vi "FPGA_main.vi"() -> ()   [LabVIEW 2016]
uses:
  <vilib>/rvi/Emulation/niFpgaGetClockAttributes.vi
  <vilib>/rvi/Emulation/niFpgaSctlEmulationGetInTimedLoop.vi
  <vilib>/rvi/Emulation/niFpgaEmulationReportErrorSimple.vi
  <vilib>/rvi/eio/common/nirviEmuTemplateMethod_errors.vi
  <vilib>/rvi/Emulation/niFpgaCriticalErrorInLSC.vi
  <vilib>/eio/EIONode/EIONode.xnode
panel:
  in  "L1":i32=52
  in  "H1":i32=48
  in  "L0":i32=80
  in  "H0":i32=20
  in  "looptime":u32=2000
  in  "Enum":enum16{"WS2812", "WS2811", "Debug"}(ring)
  in  "number of leds":i32
  in  "reset ticks)":u32=2000
  in  "color":u32
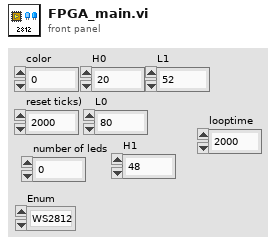
[diagram p1: front panel]
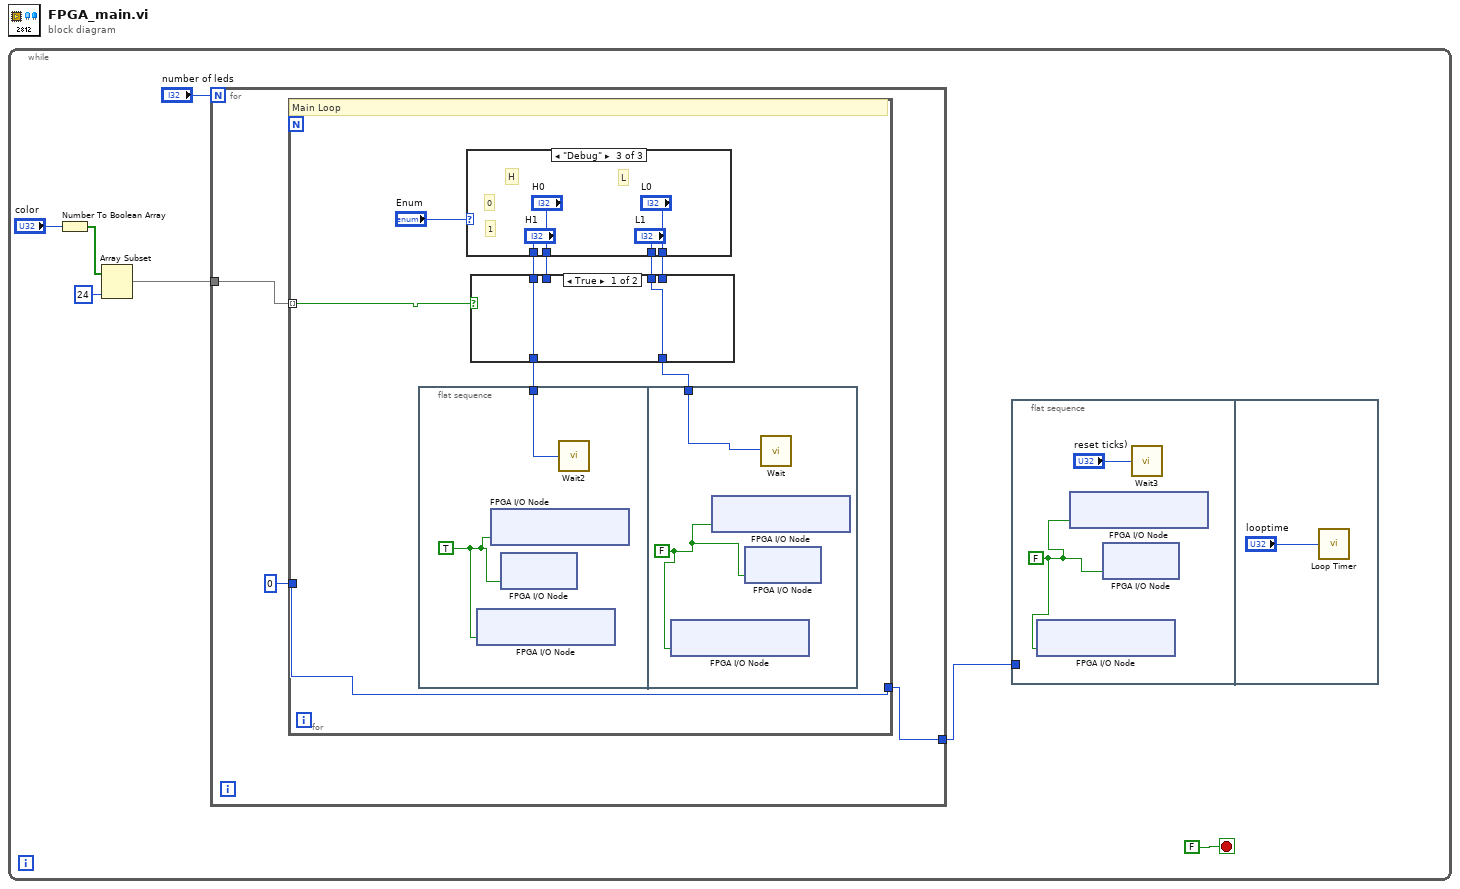
[diagram p0: block diagram]
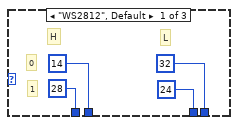
[diagram p2: hidden frame]
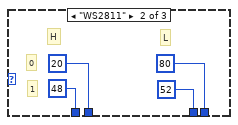
[diagram p3: hidden frame]
diagram:
  n1 = while {
    stop <- FALSE stop-if-true
    n2 = Number To Boolean Array(number="color") -> (Boolean array=w2:bool[])
    n3 = Array Subset(array=w2, length=24) -> (w3:bool[])  [unwired: 1 in]
    n4 = for {
      N: "number of leds" -> [_]
      tunnel: [w9] -> w6
      tunnel: w3 -> [w8]
      n5 = for {
        tunnel: w8 -> [w17] mode=indexing
        tunnel: [w16] -> w9
        tunnel: i16 0 -> [w16]
        # "Main Loop"
        n6 = flat-sequence {
          tunnel: w19 -> [w37]
          tunnel: w18 -> [w39]
          frame #0 {
            w36 = TRUE
            n7 = xnode "FPGA I/O Node"("ConnectorA/DIO0"=w36) -> ()  [unwired: 1 in, 1 out]
            n8 = xnode "FPGA I/O Node"("ConnectorC/DIO7"=w36) -> ()  [unwired: 1 in, 1 out]
            n9 = xnode "FPGA I/O Node"("LED0"=w36) -> ()  [unwired: 1 in, 1 out]
            n10 = call "Wait2"("Count(Ticks)"=w37) -> ()  [unwired: 1 out]
          }
          frame #1 {
            w38 = FALSE
            n11 = xnode "FPGA I/O Node"("ConnectorA/DIO0"=w38) -> ()  [unwired: 1 in, 1 out]
            n12 = xnode "FPGA I/O Node"("ConnectorC/DIO7"=w38) -> ()  [unwired: 1 in, 1 out]
            n13 = xnode "FPGA I/O Node"("LED0"=w38) -> ()  [unwired: 1 in, 1 out]
            n14 = call "Wait"("Count(Ticks)"=w39) -> ()  [unwired: 1 out]
          }
        }
        n15 = case shown="\"Debug\"" "Enum" {
          tunnel: [28 48 "H1"] -> w14
          tunnel: [14 20 "H0"] -> w13
          tunnel: [32 80 "L0"] -> w12
          tunnel: [24 52 "L1"] -> w11
          frame "WS2812", Default {
            # "L"
            # "1"
            # "0"
            # "H"
          }
          frame "WS2811" {
            # "L"
            # "1"
            # "0"
            # "H"
          }
          frame "Debug" {
            # "L"
            # "1"
            # "0"
            # "H"
          }
        }
        n16 = case shown="True" w17 {
          tunnel: [w33 w35] -> w19
          tunnel: [w32 w34] -> w18
          tunnel: w14 -> [w33 _]
          tunnel: w13 -> [_ w35]
          tunnel: w12 -> [_ w34]
          tunnel: w11 -> [w32 _]
          frame True {
          }
          frame False {
          }
        }
      }
    }
    n17 = flat-sequence {
      tunnel: w6 -> [_]
      frame #0 {
        w40 = FALSE
        n18 = xnode "FPGA I/O Node"("ConnectorA/DIO0"=w40) -> ()  [unwired: 1 in, 1 out]
        n19 = xnode "FPGA I/O Node"("ConnectorC/DIO7"=w40) -> ()  [unwired: 1 in, 1 out]
        n20 = xnode "FPGA I/O Node"("LED0"=w40) -> ()  [unwired: 1 in, 1 out]
        n21 = call "Wait3"("Count(Ticks)"="reset ticks)") -> ()  [unwired: 1 out]
      }
      frame #1 {
        n22 = call "Loop Timer"("Count(mSec)"="looptime") -> ()  [unwired: 1 out]
      }
    }
  }
